vi "ConvertFalconDriveEncoders.vi"(11 "Velocity (Raw Sensor Units per 100 ms)":i32) -> (15 "Velocity (ft/s)":dbl)   [LabVIEW 2019]
doc: "This VI converts the raw Falcon 500/Talon FX encoder postion and velocity data into units of inches and feet per second, respectively. Handles low and high gear ratios."
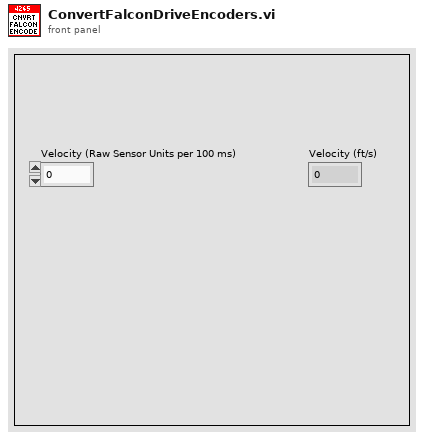
[diagram p1: front panel]
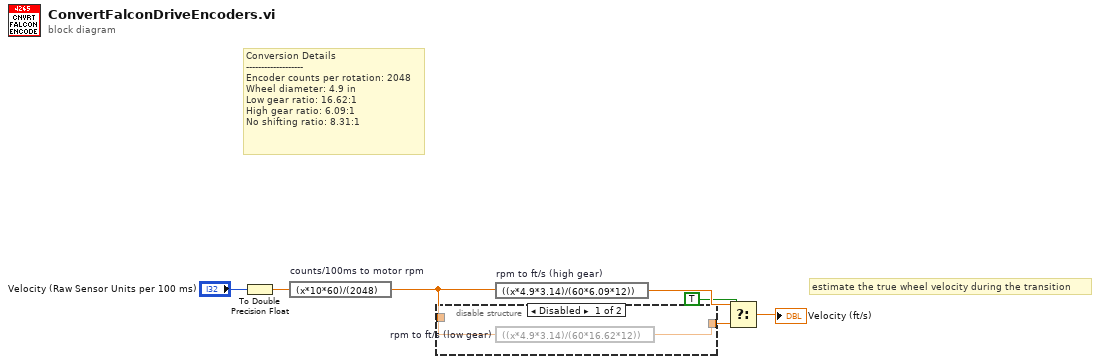
[diagram p0: block diagram]
diagram:
  # "estimate the true wheel velocity during the transition"
  # "Conversion Details\n-------------------\nEncoder counts per rotation: 2048\nWheel diameter: 4.9 in\nLow gear ratio: 16.62:1\nHigh gear ratio: 6.09:1\nNo shifting ratio: 8.31:1"
  n1 = To Double Precision Float(number="Velocity (Raw Sensor Units per 100 ms)") -> (double precision float=w7:dbl)
  n2 = expression code="(x*10*60)/(2048)" "counts/100ms to motor rpm"(w7) -> (w3:dbl)
  n3 = disable-structure shown="Disabled" {
    disable-tunnel: [w9 _] -> w5
    disable-tunnel: w3 -> [w8 _]
    frame Disabled {
      n4 = expression code="((x*4.9*3.14)/(60*16.62*12))" "rpm to ft/s (low gear)"(w8) -> (w9:dbl)
    }
    frame Enabled {
    }
  }
  n5 = expression code="((x*4.9*3.14)/(60*6.09*12))" "rpm to ft/s (high gear)"(w3) -> (w4:dbl)
  n6 = Select(t=w4, s=TRUE, f=w5) -> (s? t:f=→"Velocity (ft/s)":dbl)
